vi "data_process.vi"(0 "文件（使用对话框）":path) -> (19 "SENSOR 9":dbl[](array[numeric]), 20 "SENSOR1":dbl[](array[numeric]), 21 "SENSOR 2":dbl[](array[numeric]), 22 "SENSOR 3":dbl[](array[numeric]), 23 "SENSOR 4":dbl[](array[numeric]), 24 "SENSOR 5":dbl[](array[numeric]), 25 "SENSOR 6":dbl[](array[numeric]), 26 "SENSOR 7":dbl[](array[numeric]), 27 "SENSOR 8":dbl[](array[numeric]))   [LabVIEW 2017]
panel:
  out "PWM19":dbl[](array[numeric])
  out "PWM18":dbl[](array[numeric])
  out "PWM17":dbl[](array[numeric])
  out "PWM16":dbl[](array[numeric])
  out "PWM15":dbl[](array[numeric])
  out "PWM14":dbl[](array[numeric])
  out "PWM13":dbl[](array[numeric])
  out "PWM12":dbl[](array[numeric])
  out "PWM11":dbl[](array[numeric])
  out "PWM10":dbl[](array[numeric])
  out "PWM9":dbl[](array[numeric])
  out "PWM8":dbl[](array[numeric])
  out "PWM7":dbl[](array[numeric])
  out "PWM6":dbl[](array[numeric])
  out "PWM5":dbl[](array[numeric])
  out "PWM4":dbl[](array[numeric])
  out "PWM3":dbl[](array[numeric])
  out "匹配偏移量":i32
  out "PWM2":dbl[](array[numeric])
  out "文本":string
  out "PWM1":dbl[](array[numeric])
  # "主要功能：将9行数据分别提取出来作为一个列表"
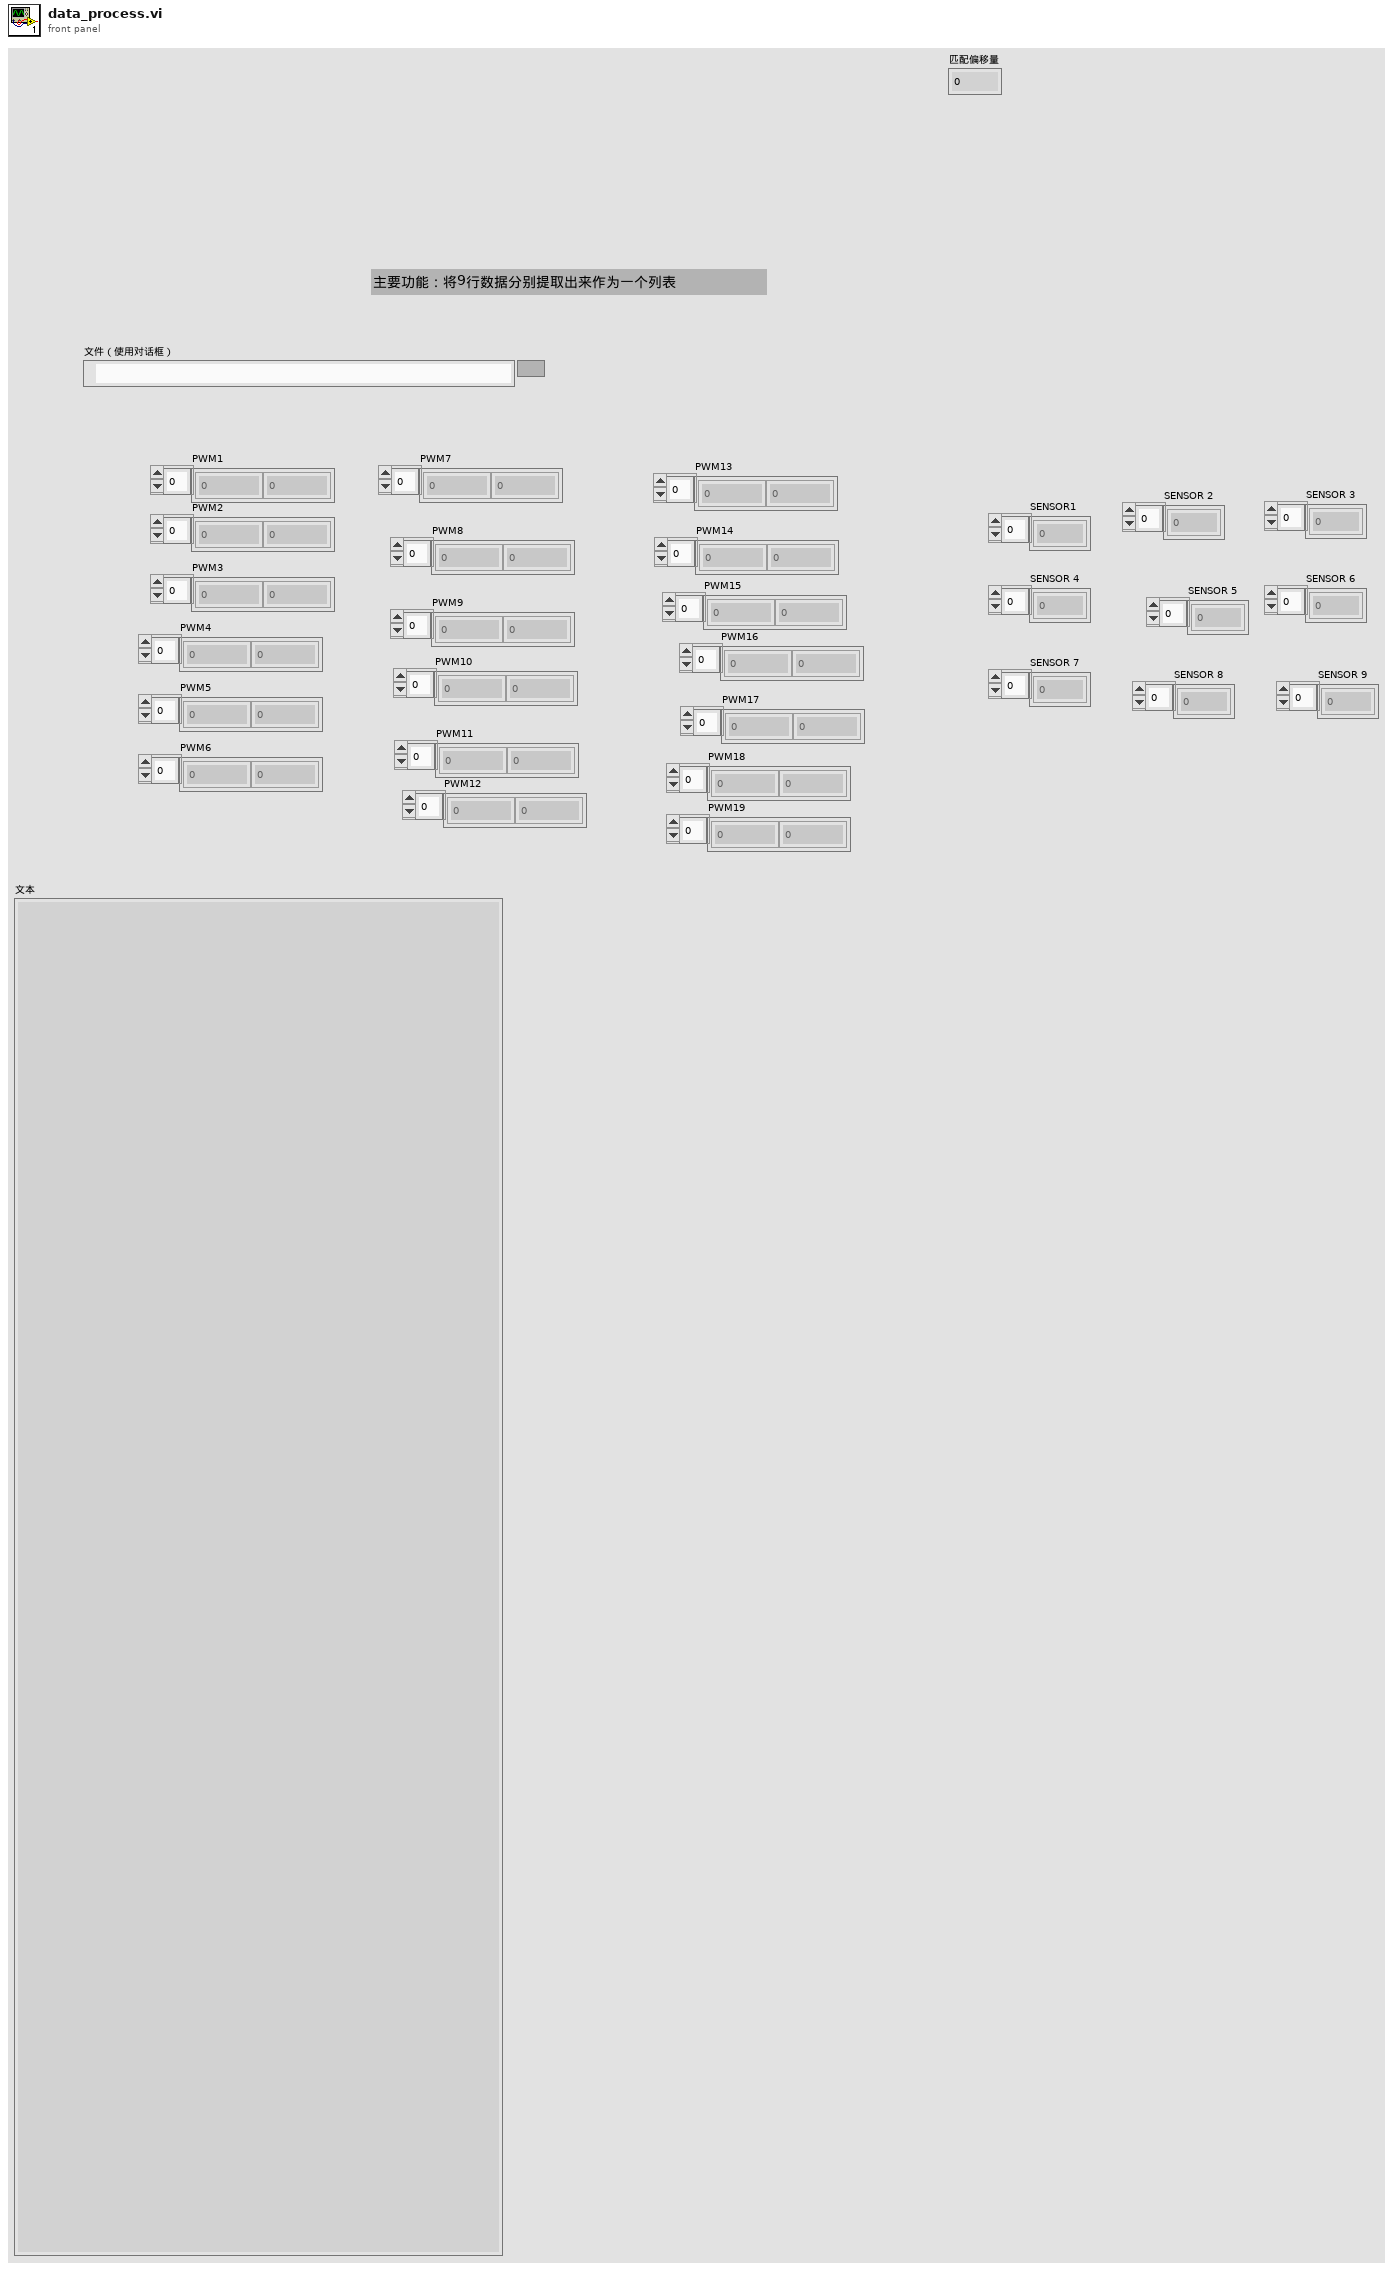
[diagram p1: front panel]
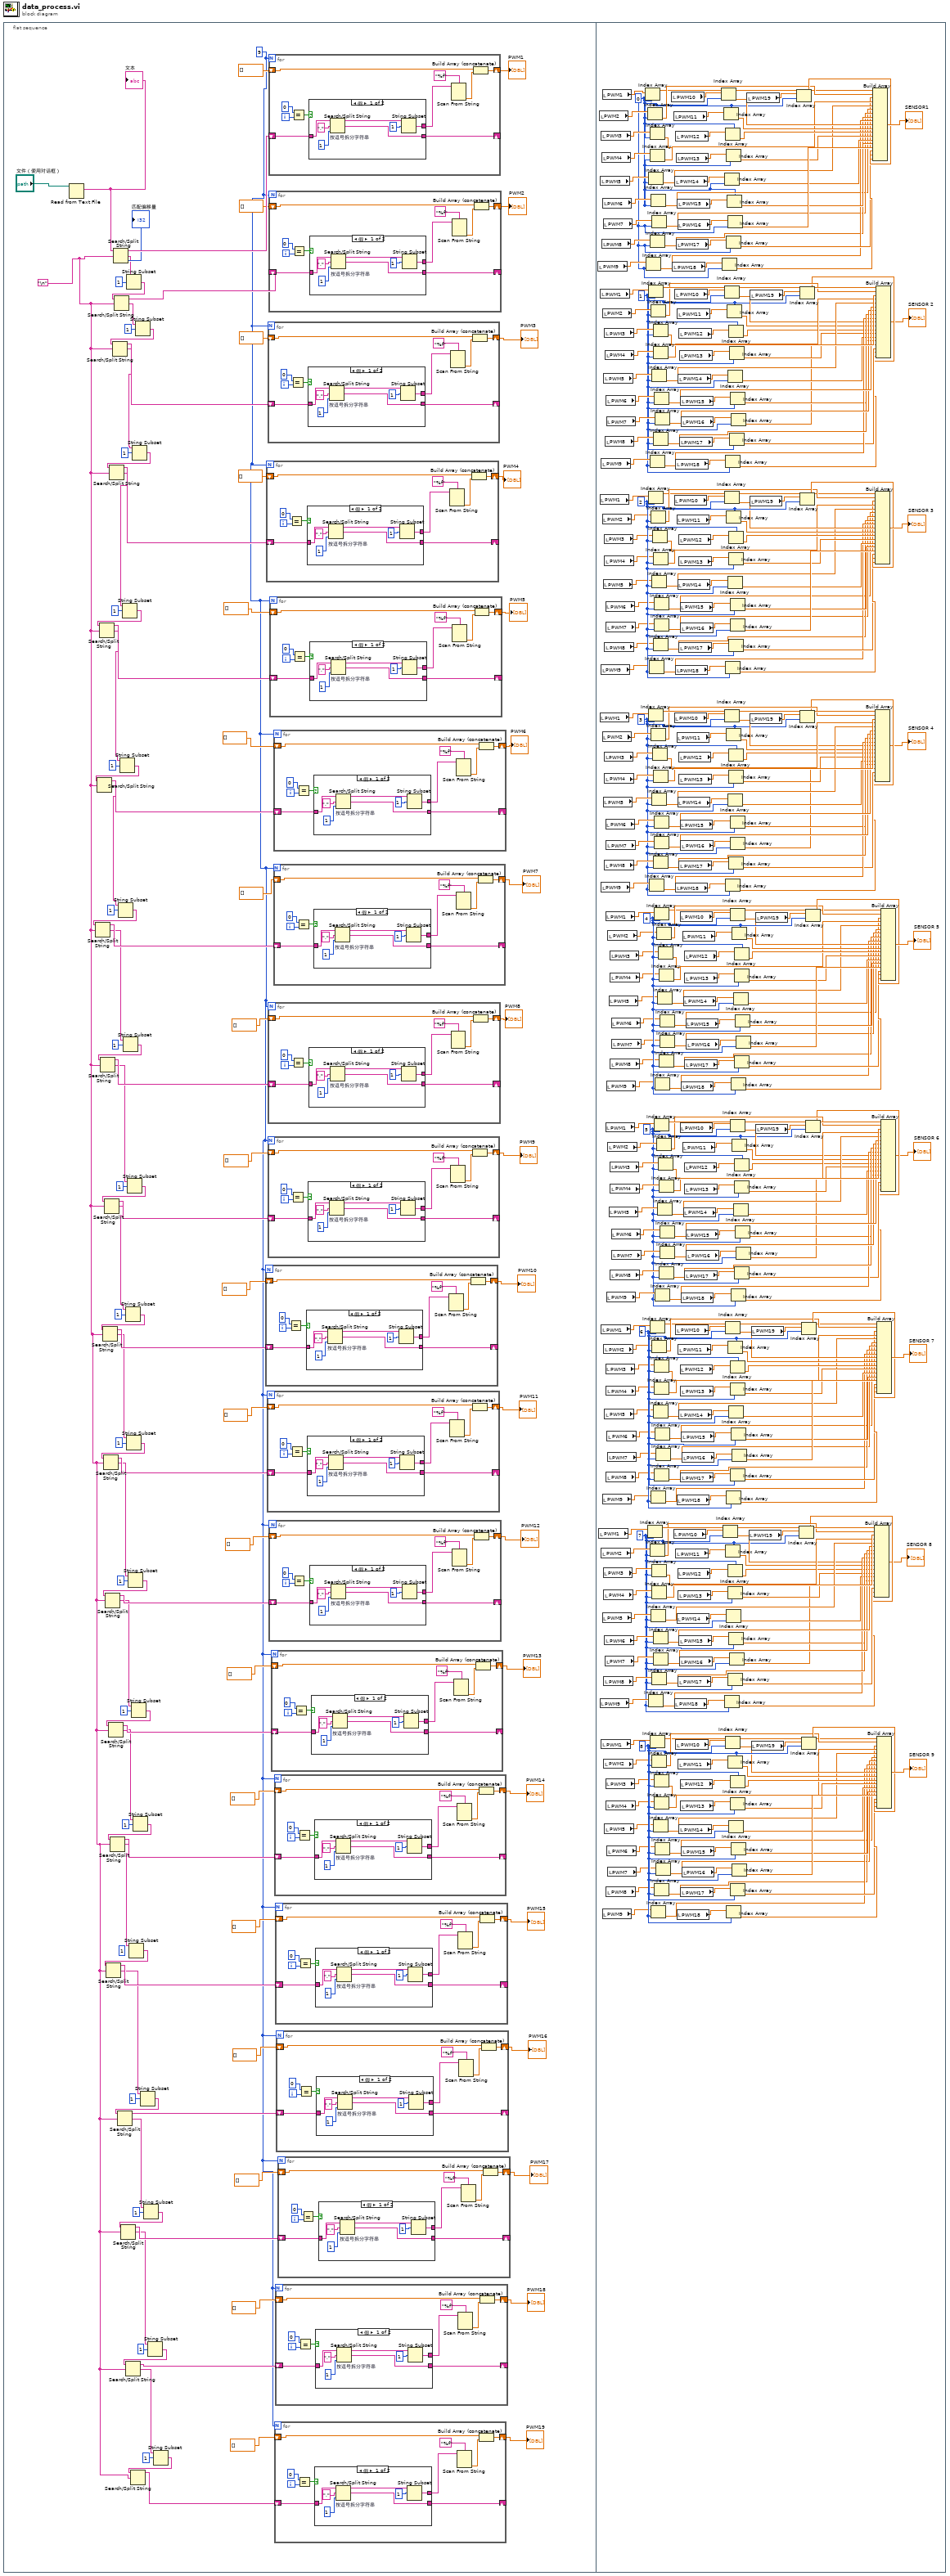
[diagram p0: block diagram]
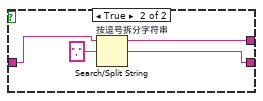
[diagram p2: hidden frame]
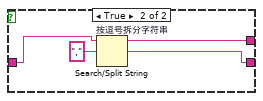
[diagram p3: hidden frame]
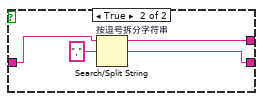
[diagram p4: hidden frame]
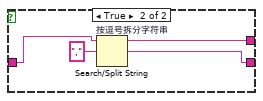
[diagram p5: hidden frame]
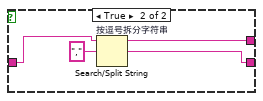
[diagram p6: hidden frame]
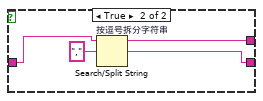
[diagram p7: hidden frame]
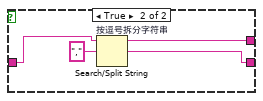
[diagram p8: hidden frame]
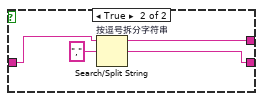
[diagram p9: hidden frame]
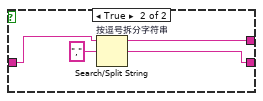
[diagram p10: hidden frame]
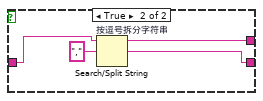
[diagram p11: hidden frame]
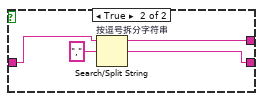
[diagram p12: hidden frame]
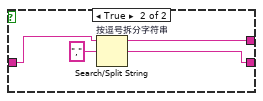
[diagram p13: hidden frame]
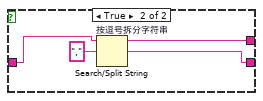
[diagram p14: hidden frame]
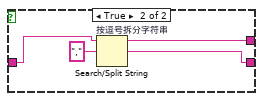
[diagram p15: hidden frame]
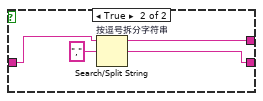
[diagram p16: hidden frame]
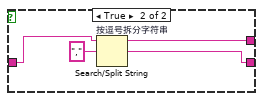
[diagram p17: hidden frame]
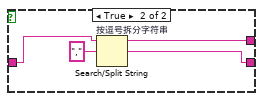
[diagram p18: hidden frame]
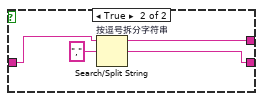
[diagram p19: hidden frame]
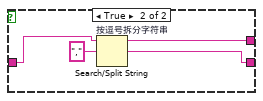
[diagram p20: hidden frame]
diagram:
  n1 = flat-sequence {
    frame #0 {
      (unwired) 1 ("偏移量(0)")
      w4 = "\n"
      w1 = 9
      n2 = Read from Text File(file (use dialog)="文件（使用对话框）") -> (text=w109:string)  [unwired: 3 in, 3 out]
      "文本" <- w109
      n3 = Search/Split String(string=w109, search string/char (-)=w4) -> (substring before match=w112:string, match + rest of string=w106:string, offset of match=→"匹配偏移量":i32)  [unwired: 1 in]
      n4 = String Subset(string=w106, offset (0)=1 ("偏移量(0)")) -> (substring=w105:string)  [unwired: 1 in]
      n5 = Search/Split String(string=w105, search string/char (-)=w4) -> (substring before match=w108:string, match + rest of string=w102:string)  [unwired: 1 in, 1 out]
      n6 = String Subset(string=w102, offset (0)=1 ("偏移量(0)")) -> (substring=w101:string)  [unwired: 1 in]
      n7 = Search/Split String(string=w101, search string/char (-)=w4) -> (substring before match=w100:string, match + rest of string=w80:string)  [unwired: 1 in, 1 out]
      n8 = String Subset(string=w80, offset (0)=1 ("偏移量(0)")) -> (substring=w84:string)  [unwired: 1 in]
      n9 = Search/Split String(string=w84, search string/char (-)=w4) -> (substring before match=w83:string, match + rest of string=w79:string)  [unwired: 1 in, 1 out]
      n10 = String Subset(string=w79, offset (0)=1 ("偏移量(0)")) -> (substring=w81:string)  [unwired: 1 in]
      n11 = Search/Split String(string=w81, search string/char (-)=w4) -> (substring before match=w78:string, match + rest of string=w75:string)  [unwired: 1 in, 1 out]
      n12 = String Subset(string=w75, offset (0)=1 ("偏移量(0)")) -> (substring=w76:string)  [unwired: 1 in]
      n13 = Search/Split String(string=w76, search string/char (-)=w4) -> (substring before match=w74:string, match + rest of string=w71:string)  [unwired: 1 in, 1 out]
      n14 = String Subset(string=w71, offset (0)=1 ("偏移量(0)")) -> (substring=w72:string)  [unwired: 1 in]
      n15 = Search/Split String(string=w72, search string/char (-)=w4) -> (substring before match=w70:string, match + rest of string=w67:string)  [unwired: 1 in, 1 out]
      n16 = String Subset(string=w67, offset (0)=1 ("偏移量(0)")) -> (substring=w68:string)  [unwired: 1 in]
      n17 = Search/Split String(string=w68, search string/char (-)=w4) -> (substring before match=w66:string, match + rest of string=w63:string)  [unwired: 1 in, 1 out]
      n18 = String Subset(string=w63, offset (0)=1 ("偏移量(0)")) -> (substring=w64:string)  [unwired: 1 in]
      n19 = Search/Split String(string=w64, search string/char (-)=w4) -> (substring before match=w62:string, match + rest of string=w40:string)  [unwired: 1 in, 1 out]
      n20 = String Subset(string=w40, offset (0)=1 ("偏移量(0)")) -> (substring=w42:string)  [unwired: 1 in]
      n21 = Search/Split String(string=w42, search string/char (-)=w4) -> (substring before match=w41:string, match + rest of string=w37:string)  [unwired: 1 in, 1 out]
      n22 = String Subset(string=w37, offset (0)=1 ("偏移量(0)")) -> (substring=w38:string)  [unwired: 1 in]
      n23 = Search/Split String(string=w38, search string/char (-)=w4) -> (substring before match=w36:string, match + rest of string=w33:string)  [unwired: 1 in, 1 out]
      n24 = String Subset(string=w33, offset (0)=1 ("偏移量(0)")) -> (substring=w34:string)  [unwired: 1 in]
      n25 = Search/Split String(string=w34, search string/char (-)=w4) -> (substring before match=w32:string, match + rest of string=w30:string)  [unwired: 1 in, 1 out]
      n26 = String Subset(string=w30, offset (0)=1 ("偏移量(0)")) -> (substring=w29:string)  [unwired: 1 in]
      n27 = Search/Split String(string=w29, search string/char (-)=w4) -> (substring before match=w26:string, match + rest of string=w25:string)  [unwired: 1 in, 1 out]
      n28 = String Subset(string=w25, offset (0)=1 ("偏移量(0)")) -> (substring=w27:string)  [unwired: 1 in]
      n29 = Search/Split String(string=w27, search string/char (-)=w4) -> (substring before match=w24:string, match + rest of string=w22:string)  [unwired: 1 in, 1 out]
      n30 = String Subset(string=w22) -> (substring=w23:string)  [unwired: 2 in]
      n31 = Search/Split String(string=w23, search string/char (-)=w4) -> (substring before match=w21:string, match + rest of string=w18:string)  [unwired: 1 in, 1 out]
      n32 = String Subset(string=w18, offset (0)=1 ("偏移量(0)")) -> (substring=w19:string)  [unwired: 1 in]
      n33 = Search/Split String(string=w19, search string/char (-)=w4) -> (substring before match=w17:string, match + rest of string=w14:string)  [unwired: 1 in, 1 out]
      n34 = String Subset(string=w14, offset (0)=1 ("偏移量(0)")) -> (substring=w15:string)  [unwired: 1 in]
      n35 = Search/Split String(string=w15, search string/char (-)=w4) -> (substring before match=w13:string, match + rest of string=w10:string)  [unwired: 1 in, 1 out]
      n36 = String Subset(string=w10, offset (0)=1 ("偏移量(0)")) -> (substring=w11:string)  [unwired: 1 in]
      n37 = Search/Split String(string=w11, search string/char (-)=w4) -> (substring before match=w9:string, match + rest of string=w3:string)  [unwired: 1 in, 1 out]
      n38 = String Subset(string=w3, offset (0)=1 ("偏移量(0)")) -> (substring=w5:string)  [unwired: 1 in]
      n39 = Search/Split String(string=w5, search string/char (-)=w4) -> (substring before match=w2:string)  [unwired: 1 in, 2 out]
      n40 = for {
        N: w1 -> [_]
        shift-right: [w310] -> _
        shift-left: w41 -> [w311]
        shift-right: [w307] -> w61
        shift-left: dbl[] [] -> [w305]
        i -> [w314]
        n41 = Equal?(x=0, y=w314) -> (x = y?=w312:bool)
        n42 = case shown="假" w312 {
          tunnel: [w320 w324] -> w310
          tunnel: w311 -> [w321 w323]
          tunnel: [w315 w322] -> w308
          frame False {
            n43 = Search/Split String "按逗号拆分字符串"(string=w321, search string/char (-)="," ("搜索字符串/字符(-)"), offset (0)=1 ("偏移量(0)")) -> (substring before match=w317:string, match + rest of string=w320:string)  [unwired: 1 out]
            n44 = String Subset(string=w317, offset (0)=1 ("偏移量(0)")) -> (substring=w315:string)  [unwired: 1 in]
          }
          frame True {
            n45 = Search/Split String "按逗号拆分字符串"(string=w323, search string/char (-)="," ("搜索字符串/字符(-)")) -> (substring before match=w322:string, match + rest of string=w324:string)  [unwired: 1 in, 1 out]
          }
        }
        n46 = Scan From String(format string="%f" ("格式字符串"), input string=w308) -> (output 1=w306:dbl)  [unwired: 3 in, 3 out]
        n47 = Build Array (concatenate)(w305, w306) -> (w307:dbl[])
      }
      "PWM10" <- w61
      n48 = for {
        N: w1 -> [_]
        shift-right: [w436] -> _
        shift-left: w83 -> [w437]
        shift-right: [w433] -> w97
        shift-left: dbl[] [] -> [w431]
        i -> [w440]
        n49 = Equal?(x=0, y=w440) -> (x = y?=w438:bool)
        n50 = case shown="假" w438 {
          tunnel: [w446 w450] -> w436
          tunnel: w437 -> [w447 w449]
          tunnel: [w441 w448] -> w434
          frame False {
            n51 = Search/Split String "按逗号拆分字符串"(string=w447, search string/char (-)="," ("搜索字符串/字符(-)"), offset (0)=1 ("偏移量(0)")) -> (substring before match=w443:string, match + rest of string=w446:string)  [unwired: 1 out]
            n52 = String Subset(string=w443, offset (0)=1 ("偏移量(0)")) -> (substring=w441:string)  [unwired: 1 in]
          }
          frame True {
            n53 = Search/Split String "按逗号拆分字符串"(string=w449, search string/char (-)="," ("搜索字符串/字符(-)")) -> (substring before match=w448:string, match + rest of string=w450:string)  [unwired: 1 in, 1 out]
          }
        }
        n54 = Scan From String(format string="%f" ("格式字符串"), input string=w434) -> (output 1=w432:dbl)  [unwired: 3 in, 3 out]
        n55 = Build Array (concatenate)(w431, w432) -> (w433:dbl[])
      }
      "PWM4" <- w97
      n56 = for {
        N: w1 -> [_]
        shift-right: [w289] -> _
        shift-left: w36 -> [w290]
        shift-right: [w286] -> w59
        shift-left: dbl[] [] -> [w284]
        i -> [w293]
        n57 = Equal?(x=0, y=w293) -> (x = y?=w291:bool)
        n58 = case shown="假" w291 {
          tunnel: [w299 w303] -> w289
          tunnel: w290 -> [w300 w302]
          tunnel: [w294 w301] -> w287
          frame False {
            n59 = Search/Split String "按逗号拆分字符串"(string=w300, search string/char (-)="," ("搜索字符串/字符(-)"), offset (0)=1 ("偏移量(0)")) -> (substring before match=w296:string, match + rest of string=w299:string)  [unwired: 1 out]
            n60 = String Subset(string=w296, offset (0)=1 ("偏移量(0)")) -> (substring=w294:string)  [unwired: 1 in]
          }
          frame True {
            n61 = Search/Split String "按逗号拆分字符串"(string=w302, search string/char (-)="," ("搜索字符串/字符(-)")) -> (substring before match=w301:string, match + rest of string=w303:string)  [unwired: 1 in, 1 out]
          }
        }
        n62 = Scan From String(format string="%f" ("格式字符串"), input string=w287) -> (output 1=w285:dbl)  [unwired: 3 in, 3 out]
        n63 = Build Array (concatenate)(w284, w285) -> (w286:dbl[])
      }
      "PWM11" <- w59
      n64 = for {
        N: w1 -> [_]
        shift-right: [w457] -> _
        shift-left: w100 -> [w458]
        shift-right: [w454] -> w98
        shift-left: dbl[] [] -> [w452]
        i -> [w461]
        n65 = Equal?(x=0, y=w461) -> (x = y?=w459:bool)
        n66 = case shown="假" w459 {
          tunnel: [w467 w471] -> w457
          tunnel: w458 -> [w468 w470]
          tunnel: [w462 w469] -> w455
          frame False {
            n67 = Search/Split String "按逗号拆分字符串"(string=w468, search string/char (-)="," ("搜索字符串/字符(-)"), offset (0)=1 ("偏移量(0)")) -> (substring before match=w464:string, match + rest of string=w467:string)  [unwired: 1 out]
            n68 = String Subset(string=w464, offset (0)=1 ("偏移量(0)")) -> (substring=w462:string)  [unwired: 1 in]
          }
          frame True {
            n69 = Search/Split String "按逗号拆分字符串"(string=w470, search string/char (-)="," ("搜索字符串/字符(-)")) -> (substring before match=w469:string, match + rest of string=w471:string)  [unwired: 1 in, 1 out]
          }
        }
        n70 = Scan From String(format string="%f" ("格式字符串"), input string=w455) -> (output 1=w453:dbl)  [unwired: 3 in, 3 out]
        n71 = Build Array (concatenate)(w452, w453) -> (w454:dbl[])
      }
      "PWM3" <- w98
      n72 = for {
        N: w1 -> [_]
        shift-right: [w331] -> _
        shift-left: w62 -> [w332]
        shift-right: [w328] -> w92
        shift-left: dbl[] [] -> [w326]
        i -> [w335]
        n73 = Equal?(x=0, y=w335) -> (x = y?=w333:bool)
        n74 = case shown="假" w333 {
          tunnel: [w341 w345] -> w331
          tunnel: w332 -> [w342 w344]
          tunnel: [w336 w343] -> w329
          frame False {
            n75 = Search/Split String "按逗号拆分字符串"(string=w342, search string/char (-)="," ("搜索字符串/字符(-)"), offset (0)=1 ("偏移量(0)")) -> (substring before match=w338:string, match + rest of string=w341:string)  [unwired: 1 out]
            n76 = String Subset(string=w338, offset (0)=1 ("偏移量(0)")) -> (substring=w336:string)  [unwired: 1 in]
          }
          frame True {
            n77 = Search/Split String "按逗号拆分字符串"(string=w344, search string/char (-)="," ("搜索字符串/字符(-)")) -> (substring before match=w343:string, match + rest of string=w345:string)  [unwired: 1 in, 1 out]
          }
        }
        n78 = Scan From String(format string="%f" ("格式字符串"), input string=w329) -> (output 1=w327:dbl)  [unwired: 3 in, 3 out]
        n79 = Build Array (concatenate)(w326, w327) -> (w328:dbl[])
      }
      "PWM9" <- w92
      n80 = for {
        N: w1 -> [_]
        shift-right: [w352] -> _
        shift-left: w66 -> [w353]
        shift-right: [w349] -> w93
        shift-left: dbl[] [] -> [w347]
        i -> [w356]
        n81 = Equal?(x=0, y=w356) -> (x = y?=w354:bool)
        n82 = case shown="假" w354 {
          tunnel: [w362 w366] -> w352
          tunnel: w353 -> [w363 w365]
          tunnel: [w357 w364] -> w350
          frame False {
            n83 = Search/Split String "按逗号拆分字符串"(string=w363, search string/char (-)="," ("搜索字符串/字符(-)"), offset (0)=1 ("偏移量(0)")) -> (substring before match=w359:string, match + rest of string=w362:string)  [unwired: 1 out]
            n84 = String Subset(string=w359, offset (0)=1 ("偏移量(0)")) -> (substring=w357:string)  [unwired: 1 in]
          }
          frame True {
            n85 = Search/Split String "按逗号拆分字符串"(string=w365, search string/char (-)="," ("搜索字符串/字符(-)")) -> (substring before match=w364:string, match + rest of string=w366:string)  [unwired: 1 in, 1 out]
          }
        }
        n86 = Scan From String(format string="%f" ("格式字符串"), input string=w350) -> (output 1=w348:dbl)  [unwired: 3 in, 3 out]
        n87 = Build Array (concatenate)(w347, w348) -> (w349:dbl[])
      }
      "PWM8" <- w93
      n88 = for {
        N: w1 -> [_]
        shift-right: [w499] -> _
        shift-left: w112 -> [w500]
        shift-right: [w496] -> w113
        shift-left: dbl[] [] -> [w494]
        i -> [w503]
        n89 = Equal?(x=0, y=w503) -> (x = y?=w501:bool)
        n90 = case shown="假" w501 {
          tunnel: [w509 w513] -> w499
          tunnel: w500 -> [w510 w512]
          tunnel: [w504 w511] -> w497
          frame False {
            n91 = Search/Split String "按逗号拆分字符串"(string=w510, search string/char (-)="," ("搜索字符串/字符(-)"), offset (0)=1 ("偏移量(0)")) -> (substring before match=w506:string, match + rest of string=w509:string)  [unwired: 1 out]
            n92 = String Subset(string=w506, offset (0)=1 ("偏移量(0)")) -> (substring=w504:string)  [unwired: 1 in]
          }
          frame True {
            n93 = Search/Split String "按逗号拆分字符串"(string=w512, search string/char (-)="," ("搜索字符串/字符(-)")) -> (substring before match=w511:string, match + rest of string=w513:string)  [unwired: 1 in, 1 out]
          }
        }
        n94 = Scan From String(format string="%f" ("格式字符串"), input string=w497) -> (output 1=w495:dbl)  [unwired: 3 in, 3 out]
        n95 = Build Array (concatenate)(w494, w495) -> (w496:dbl[])
      }
      "PWM1" <- w113
      n96 = for {
        N: w1 -> [_]
        shift-right: [w478] -> _
        shift-left: w108 -> [w479]
        shift-right: [w475] -> w110
        shift-left: dbl[] [] -> [w473]
        i -> [w482]
        n97 = Equal?(x=0, y=w482) -> (x = y?=w480:bool)
        n98 = case shown="假" w480 {
          tunnel: [w488 w492] -> w478
          tunnel: w479 -> [w489 w491]
          tunnel: [w483 w490] -> w476
          frame False {
            n99 = Search/Split String "按逗号拆分字符串"(string=w489, search string/char (-)="," ("搜索字符串/字符(-)"), offset (0)=1 ("偏移量(0)")) -> (substring before match=w485:string, match + rest of string=w488:string)  [unwired: 1 out]
            n100 = String Subset(string=w485, offset (0)=1 ("偏移量(0)")) -> (substring=w483:string)  [unwired: 1 in]
          }
          frame True {
            n101 = Search/Split String "按逗号拆分字符串"(string=w491, search string/char (-)="," ("搜索字符串/字符(-)")) -> (substring before match=w490:string, match + rest of string=w492:string)  [unwired: 1 in, 1 out]
          }
        }
        n102 = Scan From String(format string="%f" ("格式字符串"), input string=w476) -> (output 1=w474:dbl)  [unwired: 3 in, 3 out]
        n103 = Build Array (concatenate)(w473, w474) -> (w475:dbl[])
      }
      "PWM2" <- w110
      n104 = for {
        N: w1 -> [_]
        shift-right: [w268] -> _
        shift-left: w32 -> [w269]
        shift-right: [w265] -> w57
        shift-left: dbl[] [] -> [w263]
        i -> [w272]
        n105 = Equal?(x=0, y=w272) -> (x = y?=w270:bool)
        n106 = case shown="假" w270 {
          tunnel: [w278 w282] -> w268
          tunnel: w269 -> [w279 w281]
          tunnel: [w273 w280] -> w266
          frame False {
            n107 = Search/Split String "按逗号拆分字符串"(string=w279, search string/char (-)="," ("搜索字符串/字符(-)"), offset (0)=1 ("偏移量(0)")) -> (substring before match=w275:string, match + rest of string=w278:string)  [unwired: 1 out]
            n108 = String Subset(string=w275, offset (0)=1 ("偏移量(0)")) -> (substring=w273:string)  [unwired: 1 in]
          }
          frame True {
            n109 = Search/Split String "按逗号拆分字符串"(string=w281, search string/char (-)="," ("搜索字符串/字符(-)")) -> (substring before match=w280:string, match + rest of string=w282:string)  [unwired: 1 in, 1 out]
          }
        }
        n110 = Scan From String(format string="%f" ("格式字符串"), input string=w266) -> (output 1=w264:dbl)  [unwired: 3 in, 3 out]
        n111 = Build Array (concatenate)(w263, w264) -> (w265:dbl[])
      }
      "PWM12" <- w57
      n112 = for {
        N: w1 -> [_]
        shift-right: [w415] -> _
        shift-left: w78 -> [w416]
        shift-right: [w412] -> w96
        shift-left: dbl[] [] -> [w410]
        i -> [w419]
        n113 = Equal?(x=0, y=w419) -> (x = y?=w417:bool)
        n114 = case shown="假" w417 {
          tunnel: [w425 w429] -> w415
          tunnel: w416 -> [w426 w428]
          tunnel: [w420 w427] -> w413
          frame False {
            n115 = Search/Split String "按逗号拆分字符串"(string=w426, search string/char (-)="," ("搜索字符串/字符(-)"), offset (0)=1 ("偏移量(0)")) -> (substring before match=w422:string, match + rest of string=w425:string)  [unwired: 1 out]
            n116 = String Subset(string=w422, offset (0)=1 ("偏移量(0)")) -> (substring=w420:string)  [unwired: 1 in]
          }
          frame True {
            n117 = Search/Split String "按逗号拆分字符串"(string=w428, search string/char (-)="," ("搜索字符串/字符(-)")) -> (substring before match=w427:string, match + rest of string=w429:string)  [unwired: 1 in, 1 out]
          }
        }
        n118 = Scan From String(format string="%f" ("格式字符串"), input string=w413) -> (output 1=w411:dbl)  [unwired: 3 in, 3 out]
        n119 = Build Array (concatenate)(w410, w411) -> (w412:dbl[])
      }
      "PWM5" <- w96
      n120 = for {
        N: w1 -> [_]
        shift-right: [w247] -> _
        shift-left: w26 -> [w248]
        shift-right: [w244] -> w55
        shift-left: dbl[] [] -> [w242]
        i -> [w251]
        n121 = Equal?(x=0, y=w251) -> (x = y?=w249:bool)
        n122 = case shown="假" w249 {
          tunnel: [w257 w261] -> w247
          tunnel: w248 -> [w258 w260]
          tunnel: [w252 w259] -> w245
          frame False {
            n123 = Search/Split String "按逗号拆分字符串"(string=w258, search string/char (-)="," ("搜索字符串/字符(-)"), offset (0)=1 ("偏移量(0)")) -> (substring before match=w254:string, match + rest of string=w257:string)  [unwired: 1 out]
            n124 = String Subset(string=w254, offset (0)=1 ("偏移量(0)")) -> (substring=w252:string)  [unwired: 1 in]
          }
          frame True {
            n125 = Search/Split String "按逗号拆分字符串"(string=w260, search string/char (-)="," ("搜索字符串/字符(-)")) -> (substring before match=w259:string, match + rest of string=w261:string)  [unwired: 1 in, 1 out]
          }
        }
        n126 = Scan From String(format string="%f" ("格式字符串"), input string=w245) -> (output 1=w243:dbl)  [unwired: 3 in, 3 out]
        n127 = Build Array (concatenate)(w242, w243) -> (w244:dbl[])
      }
      "PWM13" <- w55
      n128 = for {
        N: w1 -> [_]
        shift-right: [w373] -> _
        shift-left: w70 -> [w374]
        shift-right: [w370] -> w94
        shift-left: dbl[] [] -> [w368]
        i -> [w377]
        n129 = Equal?(x=0, y=w377) -> (x = y?=w375:bool)
        n130 = case shown="假" w375 {
          tunnel: [w383 w387] -> w373
          tunnel: w374 -> [w384 w386]
          tunnel: [w378 w385] -> w371
          frame False {
            n131 = Search/Split String "按逗号拆分字符串"(string=w384, search string/char (-)="," ("搜索字符串/字符(-)"), offset (0)=1 ("偏移量(0)")) -> (substring before match=w380:string, match + rest of string=w383:string)  [unwired: 1 out]
            n132 = String Subset(string=w380, offset (0)=1 ("偏移量(0)")) -> (substring=w378:string)  [unwired: 1 in]
          }
          frame True {
            n133 = Search/Split String "按逗号拆分字符串"(string=w386, search string/char (-)="," ("搜索字符串/字符(-)")) -> (substring before match=w385:string, match + rest of string=w387:string)  [unwired: 1 in, 1 out]
          }
        }
        n134 = Scan From String(format string="%f" ("格式字符串"), input string=w371) -> (output 1=w369:dbl)  [unwired: 3 in, 3 out]
        n135 = Build Array (concatenate)(w368, w369) -> (w370:dbl[])
      }
      "PWM7" <- w94
      n136 = for {
        N: w1 -> [_]
        shift-right: [w394] -> _
        shift-left: w74 -> [w395]
        shift-right: [w391] -> w95
        shift-left: dbl[] [] -> [w389]
        i -> [w398]
        n137 = Equal?(x=0, y=w398) -> (x = y?=w396:bool)
        n138 = case shown="假" w396 {
          tunnel: [w404 w408] -> w394
          tunnel: w395 -> [w405 w407]
          tunnel: [w399 w406] -> w392
          frame False {
            n139 = Search/Split String "按逗号拆分字符串"(string=w405, search string/char (-)="," ("搜索字符串/字符(-)"), offset (0)=1 ("偏移量(0)")) -> (substring before match=w401:string, match + rest of string=w404:string)  [unwired: 1 out]
            n140 = String Subset(string=w401, offset (0)=1 ("偏移量(0)")) -> (substring=w399:string)  [unwired: 1 in]
          }
          frame True {
            n141 = Search/Split String "按逗号拆分字符串"(string=w407, search string/char (-)="," ("搜索字符串/字符(-)")) -> (substring before match=w406:string, match + rest of string=w408:string)  [unwired: 1 in, 1 out]
          }
        }
        n142 = Scan From String(format string="%f" ("格式字符串"), input string=w392) -> (output 1=w390:dbl)  [unwired: 3 in, 3 out]
        n143 = Build Array (concatenate)(w389, w390) -> (w391:dbl[])
      }
      "PWM6" <- w95
      n144 = for {
        N: w1 -> [_]
        shift-right: [w226] -> _
        shift-left: w24 -> [w227]
        shift-right: [w223] -> w53
        shift-left: dbl[] [] -> [w221]
        i -> [w230]
        n145 = Equal?(x=0, y=w230) -> (x = y?=w228:bool)
        n146 = case shown="假" w228 {
          tunnel: [w236 w240] -> w226
          tunnel: w227 -> [w237 w239]
          tunnel: [w231 w238] -> w224
          frame False {
            n147 = Search/Split String "按逗号拆分字符串"(string=w237, search string/char (-)="," ("搜索字符串/字符(-)"), offset (0)=1 ("偏移量(0)")) -> (substring before match=w233:string, match + rest of string=w236:string)  [unwired: 1 out]
            n148 = String Subset(string=w233, offset (0)=1 ("偏移量(0)")) -> (substring=w231:string)  [unwired: 1 in]
          }
          frame True {
            n149 = Search/Split String "按逗号拆分字符串"(string=w239, search string/char (-)="," ("搜索字符串/字符(-)")) -> (substring before match=w238:string, match + rest of string=w240:string)  [unwired: 1 in, 1 out]
          }
        }
        n150 = Scan From String(format string="%f" ("格式字符串"), input string=w224) -> (output 1=w222:dbl)  [unwired: 3 in, 3 out]
        n151 = Build Array (concatenate)(w221, w222) -> (w223:dbl[])
      }
      "PWM14" <- w53
      n152 = for {
        N: w1 -> [_]
        shift-right: [w121] -> _
        shift-left: w2 -> [w122]
        shift-right: [w118] -> w8
        shift-left: dbl[] [] -> [w116]
        i -> [w125]
        n153 = Equal?(x=0, y=w125) -> (x = y?=w123:bool)
        n154 = case shown="假" w123 {
          tunnel: [w131 w135] -> w121
          tunnel: w122 -> [w132 w134]
          tunnel: [w126 w133] -> w119
          frame False {
            n155 = Search/Split String "按逗号拆分字符串"(string=w132, search string/char (-)="," ("搜索字符串/字符(-)"), offset (0)=1 ("偏移量(0)")) -> (substring before match=w128:string, match + rest of string=w131:string)  [unwired: 1 out]
            n156 = String Subset(string=w128, offset (0)=1 ("偏移量(0)")) -> (substring=w126:string)  [unwired: 1 in]
          }
          frame True {
            n157 = Search/Split String "按逗号拆分字符串"(string=w134, search string/char (-)="," ("搜索字符串/字符(-)")) -> (substring before match=w133:string, match + rest of string=w135:string)  [unwired: 1 in, 1 out]
          }
        }
        n158 = Scan From String(format string="%f" ("格式字符串"), input string=w119) -> (output 1=w117:dbl)  [unwired: 3 in, 3 out]
        n159 = Build Array (concatenate)(w116, w117) -> (w118:dbl[])
      }
      "PWM19" <- w8
      n160 = for {
        N: w1 -> [_]
        shift-right: [w205] -> _
        shift-left: w21 -> [w206]
        shift-right: [w202] -> w51
        shift-left: dbl[] [] -> [w200]
        i -> [w209]
        n161 = Equal?(x=0, y=w209) -> (x = y?=w207:bool)
        n162 = case shown="假" w207 {
          tunnel: [w215 w219] -> w205
          tunnel: w206 -> [w216 w218]
          tunnel: [w210 w217] -> w203
          frame False {
            n163 = Search/Split String "按逗号拆分字符串"(string=w216, search string/char (-)="," ("搜索字符串/字符(-)"), offset (0)=1 ("偏移量(0)")) -> (substring before match=w212:string, match + rest of string=w215:string)  [unwired: 1 out]
            n164 = String Subset(string=w212, offset (0)=1 ("偏移量(0)")) -> (substring=w210:string)  [unwired: 1 in]
          }
          frame True {
            n165 = Search/Split String "按逗号拆分字符串"(string=w218, search string/char (-)="," ("搜索字符串/字符(-)")) -> (substring before match=w217:string, match + rest of string=w219:string)  [unwired: 1 in, 1 out]
          }
        }
        n166 = Scan From String(format string="%f" ("格式字符串"), input string=w203) -> (output 1=w201:dbl)  [unwired: 3 in, 3 out]
        n167 = Build Array (concatenate)(w200, w201) -> (w202:dbl[])
      }
      "PWM15" <- w51
      n168 = for {
        N: w1 -> [_]
        shift-right: [w142] -> _
        shift-left: w9 -> [w143]
        shift-right: [w139] -> w45
        shift-left: dbl[] [] -> [w137]
        i -> [w146]
        n169 = Equal?(x=0, y=w146) -> (x = y?=w144:bool)
        n170 = case shown="假" w144 {
          tunnel: [w152 w156] -> w142
          tunnel: w143 -> [w153 w155]
          tunnel: [w147 w154] -> w140
          frame False {
            n171 = Search/Split String "按逗号拆分字符串"(string=w153, search string/char (-)="," ("搜索字符串/字符(-)"), offset (0)=1 ("偏移量(0)")) -> (substring before match=w149:string, match + rest of string=w152:string)  [unwired: 1 out]
            n172 = String Subset(string=w149, offset (0)=1 ("偏移量(0)")) -> (substring=w147:string)  [unwired: 1 in]
          }
          frame True {
            n173 = Search/Split String "按逗号拆分字符串"(string=w155, search string/char (-)="," ("搜索字符串/字符(-)")) -> (substring before match=w154:string, match + rest of string=w156:string)  [unwired: 1 in, 1 out]
          }
        }
        n174 = Scan From String(format string="%f" ("格式字符串"), input string=w140) -> (output 1=w138:dbl)  [unwired: 3 in, 3 out]
        n175 = Build Array (concatenate)(w137, w138) -> (w139:dbl[])
      }
      "PWM18" <- w45
      n176 = for {
        N: w1 -> [_]
        shift-right: [w184] -> _
        shift-left: w17 -> [w185]
        shift-right: [w181] -> w49
        shift-left: dbl[] [] -> [w179]
        i -> [w188]
        n177 = Equal?(x=0, y=w188) -> (x = y?=w186:bool)
        n178 = case shown="假" w186 {
          tunnel: [w194 w198] -> w184
          tunnel: w185 -> [w195 w197]
          tunnel: [w189 w196] -> w182
          frame False {
            n179 = Search/Split String "按逗号拆分字符串"(string=w195, search string/char (-)="," ("搜索字符串/字符(-)"), offset (0)=1 ("偏移量(0)")) -> (substring before match=w191:string, match + rest of string=w194:string)  [unwired: 1 out]
            n180 = String Subset(string=w191, offset (0)=1 ("偏移量(0)")) -> (substring=w189:string)  [unwired: 1 in]
          }
          frame True {
            n181 = Search/Split String "按逗号拆分字符串"(string=w197, search string/char (-)="," ("搜索字符串/字符(-)")) -> (substring before match=w196:string, match + rest of string=w198:string)  [unwired: 1 in, 1 out]
          }
        }
        n182 = Scan From String(format string="%f" ("格式字符串"), input string=w182) -> (output 1=w180:dbl)  [unwired: 3 in, 3 out]
        n183 = Build Array (concatenate)(w179, w180) -> (w181:dbl[])
      }
      "PWM16" <- w49
      n184 = for {
        N: w1 -> [_]
        shift-right: [w163] -> _
        shift-left: w13 -> [w164]
        shift-right: [w160] -> w47
        shift-left: dbl[] [] -> [w158]
        i -> [w167]
        n185 = Equal?(x=0, y=w167) -> (x = y?=w165:bool)
        n186 = case shown="假" w165 {
          tunnel: [w173 w177] -> w163
          tunnel: w164 -> [w174 w176]
          tunnel: [w168 w175] -> w161
          frame False {
            n187 = Search/Split String "按逗号拆分字符串"(string=w174, search string/char (-)="," ("搜索字符串/字符(-)"), offset (0)=1 ("偏移量(0)")) -> (substring before match=w170:string, match + rest of string=w173:string)  [unwired: 1 out]
            n188 = String Subset(string=w170, offset (0)=1 ("偏移量(0)")) -> (substring=w168:string)  [unwired: 1 in]
          }
          frame True {
            n189 = Search/Split String "按逗号拆分字符串"(string=w176, search string/char (-)="," ("搜索字符串/字符(-)")) -> (substring before match=w175:string, match + rest of string=w177:string)  [unwired: 1 in, 1 out]
          }
        }
        n190 = Scan From String(format string="%f" ("格式字符串"), input string=w161) -> (output 1=w159:dbl)  [unwired: 3 in, 3 out]
        n191 = Build Array (concatenate)(w158, w159) -> (w160:dbl[])
      }
      "PWM17" <- w47
    }
    frame #1 {
      w554 = 8 ("索引")
      w555 = 7 ("索引")
      w634 = 6 ("索引")
      w635 = 5 ("索引")
      w714 = 4 ("索引")
      w715 = 3 ("索引")
      w794 = 2 ("索引")
      w796 = 1 ("索引")
      w795 = 0 ("索引")
      n192 = local read "PWM9"() -> (w805:dbl[])
      n193 = local read "PWM1"() -> (w594:dbl[])
      n194 = local read "PWM2"() -> (w798:dbl[])
      n195 = local read "PWM1"() -> (w755:dbl[])
      n196 = local read "PWM1"() -> (w754:dbl[])
      n197 = local read "PWM9"() -> (w585:dbl[])
      n198 = local read "PWM5"() -> (w801:dbl[])
      n199 = local read "PWM1"() -> (w873:dbl[])
      n200 = local read "PWM9"() -> (w764:dbl[])
      n201 = local read "PWM9"() -> (w745:dbl[])
      n202 = local read "PWM3"() -> (w799:dbl[])
      n203 = local read "PWM9"() -> (w864:dbl[])
      n204 = local read "PWM1"() -> (w595:dbl[])
      n205 = local read "PWM2"() -> (w592:dbl[])
      n206 = local read "PWM1"() -> (w515:dbl[])
      n207 = local read "PWM4"() -> (w800:dbl[])
      n208 = local read "PWM8"() -> (w804:dbl[])
      n209 = local read "PWM1"() -> (w874:dbl[])
      n210 = local read "PWM2"() -> (w757:dbl[])
      n211 = local read "PWM2"() -> (w752:dbl[])
      n212 = local read "PWM9"() -> (w604:dbl[])
      n213 = local read "PWM5"() -> (w589:dbl[])
      n214 = local read "PWM9"() -> (w524:dbl[])
      n215 = local read "PWM6"() -> (w802:dbl[])
      n216 = local read "PWM2"() -> (w871:dbl[])
      n217 = local read "PWM7"() -> (w803:dbl[])
      n218 = local read "PWM5"() -> (w760:dbl[])
      n219 = local read "PWM5"() -> (w749:dbl[])
      n220 = local read "PWM3"() -> (w591:dbl[])
      n221 = local read "PWM5"() -> (w868:dbl[])
      n222 = local read "PWM2"() -> (w597:dbl[])
      n223 = local read "PWM4"() -> (w590:dbl[])
      n224 = local read "PWM8"() -> (w586:dbl[])
      n225 = local read "PWM2"() -> (w517:dbl[])
      n226 = local read "PWM3"() -> (w758:dbl[])
      n227 = local read "PWM3"() -> (w751:dbl[])
      n228 = local read "PWM3"() -> (w870:dbl[])
      n229 = local read "PWM4"() -> (w759:dbl[])
      n230 = local read "PWM8"() -> (w763:dbl[])
      n231 = local read "PWM4"() -> (w750:dbl[])
      n232 = local read "PWM8"() -> (w746:dbl[])
      n233 = local read "PWM5"() -> (w600:dbl[])
      n234 = local read "PWM6"() -> (w588:dbl[])
      n235 = local read "PWM5"() -> (w520:dbl[])
      n236 = local read "PWM4"() -> (w869:dbl[])
      n237 = local read "PWM8"() -> (w865:dbl[])
      n238 = local read "PWM7"() -> (w587:dbl[])
      n239 = local read "PWM6"() -> (w761:dbl[])
      n240 = local read "PWM6"() -> (w748:dbl[])
      n241 = local read "PWM1"() -> (w675:dbl[])
      n242 = local read "PWM1"() -> (w674:dbl[])
      n243 = local read "PWM3"() -> (w598:dbl[])
      n244 = local read "PWM3"() -> (w518:dbl[])
      n245 = local read "PWM6"() -> (w867:dbl[])
      n246 = local read "PWM7"() -> (w762:dbl[])
      n247 = local read "PWM7"() -> (w747:dbl[])
      n248 = local read "PWM4"() -> (w599:dbl[])
      n249 = local read "PWM8"() -> (w603:dbl[])
      n250 = local read "PWM4"() -> (w519:dbl[])
      n251 = local read "PWM8"() -> (w523:dbl[])
      n252 = local read "PWM7"() -> (w866:dbl[])
      n253 = local read "PWM9"() -> (w684:dbl[])
      n254 = local read "PWM9"() -> (w665:dbl[])
      n255 = local read "PWM6"() -> (w601:dbl[])
      n256 = local read "PWM6"() -> (w521:dbl[])
      n257 = local read "PWM7"() -> (w602:dbl[])
      n258 = local read "PWM7"() -> (w522:dbl[])
      n259 = local read "PWM2"() -> (w677:dbl[])
      n260 = local read "PWM2"() -> (w672:dbl[])
      n261 = local read "PWM5"() -> (w680:dbl[])
      n262 = local read "PWM5"() -> (w669:dbl[])
      n263 = local read "PWM3"() -> (w678:dbl[])
      n264 = local read "PWM3"() -> (w671:dbl[])
      n265 = local read "PWM4"() -> (w679:dbl[])
      n266 = local read "PWM8"() -> (w683:dbl[])
      n267 = local read "PWM4"() -> (w670:dbl[])
      n268 = local read "PWM8"() -> (w666:dbl[])
      n269 = local read "PWM6"() -> (w681:dbl[])
      n270 = local read "PWM6"() -> (w668:dbl[])
      n271 = local read "PWM7"() -> (w682:dbl[])
      n272 = local read "PWM7"() -> (w667:dbl[])
      n273 = Index Array(array=w874, index=w795) -> (element=w797:dbl)
      n274 = Index Array(array=w805, index=w795) -> (element=w823:dbl)
      n275 = Index Array(array=w594, index=w555) -> (element=w593:dbl)
      n276 = Index Array(array=w798, index=w795) -> (element=w816:dbl)
      n277 = Index Array(array=w755, index=w794) -> (element=w756:dbl)
      n278 = Index Array(array=w754, index=w715) -> (element=w753:dbl)
      n279 = Index Array(array=w585, index=w555) -> (element=w567:dbl)
      n280 = Index Array(array=w801, index=w795) -> (element=w819:dbl)
      n281 = Index Array(array=w873, index=w796) -> (element=w872:dbl)
      n282 = Index Array(array=w764, index=w794) -> (element=w782:dbl)
      n283 = Index Array(array=w745, index=w715) -> (element=w727:dbl)
      n284 = Index Array(array=w799, index=w795) -> (element=w817:dbl)
      n285 = Index Array(array=w864, index=w796) -> (element=w846:dbl)
      n286 = Index Array(array=w595, index=w634) -> (element=w596:dbl)
      n287 = Index Array(array=w592, index=w555) -> (element=w574:dbl)
      n288 = Index Array(array=w515, index=w554) -> (element=w516:dbl)
      n289 = Index Array(array=w800, index=w795) -> (element=w818:dbl)
      n290 = Index Array(array=w804, index=w795) -> (element=w822:dbl)
      n291 = Index Array(array=w757, index=w794) -> (element=w775:dbl)
      n292 = Index Array(array=w752, index=w715) -> (element=w734:dbl)
      n293 = Index Array(array=w604, index=w634) -> (element=w622:dbl)
      n294 = Index Array(array=w589, index=w555) -> (element=w571:dbl)
      n295 = Index Array(array=w524, index=w554) -> (element=w542:dbl)
      n296 = Index Array(array=w802, index=w795) -> (element=w820:dbl)
      n297 = Index Array(array=w871, index=w796) -> (element=w853:dbl)
      n298 = Index Array(array=w803, index=w795) -> (element=w821:dbl)
      n299 = Index Array(array=w760, index=w794) -> (element=w778:dbl)
      n300 = Index Array(array=w749, index=w715) -> (element=w731:dbl)
      n301 = Index Array(array=w591, index=w555) -> (element=w573:dbl)
      n302 = Index Array(array=w868, index=w796) -> (element=w850:dbl)
      n303 = Index Array(array=w597, index=w634) -> (element=w615:dbl)
      n304 = Index Array(array=w590, index=w555) -> (element=w572:dbl)
      n305 = Index Array(array=w586, index=w555) -> (element=w568:dbl)
      n306 = Index Array(array=w517, index=w554) -> (element=w535:dbl)
      n307 = Index Array(array=w758, index=w794) -> (element=w776:dbl)
      n308 = Index Array(array=w751, index=w715) -> (element=w733:dbl)
      n309 = Index Array(array=w870, index=w796) -> (element=w852:dbl)
      n310 = Index Array(array=w759, index=w794) -> (element=w777:dbl)
      n311 = Index Array(array=w763, index=w794) -> (element=w781:dbl)
      n312 = Index Array(array=w750, index=w715) -> (element=w732:dbl)
      n313 = Index Array(array=w746, index=w715) -> (element=w728:dbl)
      n314 = Index Array(array=w600, index=w634) -> (element=w618:dbl)
      n315 = Index Array(array=w588, index=w555) -> (element=w570:dbl)
      n316 = Index Array(array=w520, index=w554) -> (element=w538:dbl)
      n317 = Index Array(array=w869, index=w796) -> (element=w851:dbl)
      n318 = Index Array(array=w865, index=w796) -> (element=w847:dbl)
      n319 = Index Array(array=w587, index=w555) -> (element=w569:dbl)
      n320 = Index Array(array=w761, index=w794) -> (element=w779:dbl)
      n321 = Index Array(array=w748, index=w715) -> (element=w730:dbl)
      n322 = Index Array(array=w675, index=w714) -> (element=w676:dbl)
      n323 = Index Array(array=w674, index=w635) -> (element=w673:dbl)
      n324 = Index Array(array=w598, index=w634) -> (element=w616:dbl)
      n325 = Index Array(array=w518, index=w554) -> (element=w536:dbl)
      n326 = Index Array(array=w867, index=w796) -> (element=w849:dbl)
      n327 = Index Array(array=w762, index=w794) -> (element=w780:dbl)
      n328 = Index Array(array=w747, index=w715) -> (element=w729:dbl)
      n329 = Index Array(array=w599, index=w634) -> (element=w617:dbl)
      n330 = Index Array(array=w603, index=w634) -> (element=w621:dbl)
      n331 = Index Array(array=w519, index=w554) -> (element=w537:dbl)
      n332 = Index Array(array=w523, index=w554) -> (element=w541:dbl)
      n333 = Index Array(array=w866, index=w796) -> (element=w848:dbl)
      n334 = Index Array(array=w684, index=w714) -> (element=w702:dbl)
      n335 = Index Array(array=w665, index=w635) -> (element=w647:dbl)
      n336 = Index Array(array=w601, index=w634) -> (element=w619:dbl)
      n337 = Index Array(array=w521, index=w554) -> (element=w539:dbl)
      n338 = Index Array(array=w602, index=w634) -> (element=w620:dbl)
      n339 = Index Array(array=w522, index=w554) -> (element=w540:dbl)
      n340 = Index Array(array=w677, index=w714) -> (element=w695:dbl)
      n341 = Index Array(array=w672, index=w635) -> (element=w654:dbl)
      n342 = Index Array(array=w680, index=w714) -> (element=w698:dbl)
      n343 = Index Array(array=w669, index=w635) -> (element=w651:dbl)
      n344 = Index Array(array=w678, index=w714) -> (element=w696:dbl)
      n345 = Index Array(array=w671, index=w635) -> (element=w653:dbl)
      n346 = Index Array(array=w679, index=w714) -> (element=w697:dbl)
      n347 = Index Array(array=w683, index=w714) -> (element=w701:dbl)
      n348 = Index Array(array=w670, index=w635) -> (element=w652:dbl)
      n349 = Index Array(array=w666, index=w635) -> (element=w648:dbl)
      n350 = Index Array(array=w681, index=w714) -> (element=w699:dbl)
      n351 = Index Array(array=w668, index=w635) -> (element=w650:dbl)
      n352 = Index Array(array=w682, index=w714) -> (element=w700:dbl)
      n353 = Index Array(array=w667, index=w635) -> (element=w649:dbl)
      n354 = local read "PWM10"() -> (w814:dbl[])
      n355 = local read "PWM18"() -> (w806:dbl[])
      n356 = local read "PWM10"() -> (w576:dbl[])
      n357 = local read "PWM11"() -> (w813:dbl[])
      n358 = local read "PWM10"() -> (w773:dbl[])
      n359 = local read "PWM10"() -> (w736:dbl[])
      n360 = local read "PWM18"() -> (w584:dbl[])
      n361 = local read "PWM14"() -> (w810:dbl[])
      n362 = local read "PWM10"() -> (w855:dbl[])
      n363 = local read "PWM18"() -> (w765:dbl[])
      n364 = local read "PWM18"() -> (w744:dbl[])
      n365 = local read "PWM12"() -> (w812:dbl[])
      n366 = local read "PWM18"() -> (w863:dbl[])
      n367 = local read "PWM10"() -> (w613:dbl[])
      n368 = local read "PWM11"() -> (w577:dbl[])
      n369 = local read "PWM10"() -> (w533:dbl[])
      n370 = local read "PWM13"() -> (w811:dbl[])
      n371 = local read "PWM17"() -> (w807:dbl[])
      n372 = local read "PWM11"() -> (w772:dbl[])
      n373 = local read "PWM11"() -> (w737:dbl[])
      n374 = local read "PWM18"() -> (w605:dbl[])
      n375 = local read "PWM14"() -> (w580:dbl[])
      n376 = local read "PWM18"() -> (w525:dbl[])
      n377 = local read "PWM15"() -> (w809:dbl[])
      n378 = local read "PWM11"() -> (w856:dbl[])
      n379 = local read "PWM16"() -> (w808:dbl[])
      n380 = local read "PWM14"() -> (w769:dbl[])
      n381 = local read "PWM14"() -> (w740:dbl[])
      n382 = local read "PWM12"() -> (w578:dbl[])
      n383 = local read "PWM14"() -> (w859:dbl[])
      n384 = local read "PWM11"() -> (w612:dbl[])
      n385 = local read "PWM13"() -> (w579:dbl[])
      n386 = local read "PWM17"() -> (w583:dbl[])
      n387 = local read "PWM11"() -> (w532:dbl[])
      n388 = local read "PWM12"() -> (w771:dbl[])
      n389 = local read "PWM12"() -> (w738:dbl[])
      n390 = local read "PWM12"() -> (w857:dbl[])
      n391 = local read "PWM13"() -> (w770:dbl[])
      n392 = local read "PWM17"() -> (w766:dbl[])
      n393 = local read "PWM13"() -> (w739:dbl[])
      n394 = local read "PWM17"() -> (w743:dbl[])
      n395 = local read "PWM14"() -> (w609:dbl[])
      n396 = local read "PWM15"() -> (w581:dbl[])
      n397 = local read "PWM14"() -> (w529:dbl[])
      n398 = local read "PWM13"() -> (w858:dbl[])
      n399 = local read "PWM17"() -> (w862:dbl[])
      n400 = local read "PWM16"() -> (w582:dbl[])
      n401 = local read "PWM15"() -> (w768:dbl[])
      n402 = local read "PWM15"() -> (w741:dbl[])
      n403 = local read "PWM10"() -> (w693:dbl[])
      n404 = local read "PWM10"() -> (w656:dbl[])
      n405 = local read "PWM12"() -> (w611:dbl[])
      n406 = local read "PWM12"() -> (w531:dbl[])
      n407 = local read "PWM15"() -> (w860:dbl[])
      n408 = local read "PWM16"() -> (w767:dbl[])
      n409 = local read "PWM16"() -> (w742:dbl[])
      n410 = local read "PWM13"() -> (w610:dbl[])
      n411 = local read "PWM17"() -> (w606:dbl[])
      n412 = local read "PWM13"() -> (w530:dbl[])
      n413 = local read "PWM17"() -> (w526:dbl[])
      n414 = local read "PWM16"() -> (w861:dbl[])
      n415 = local read "PWM18"() -> (w685:dbl[])
      n416 = local read "PWM18"() -> (w664:dbl[])
      n417 = local read "PWM15"() -> (w608:dbl[])
      n418 = local read "PWM15"() -> (w528:dbl[])
      n419 = local read "PWM16"() -> (w607:dbl[])
      n420 = local read "PWM16"() -> (w527:dbl[])
      n421 = local read "PWM11"() -> (w692:dbl[])
      n422 = local read "PWM11"() -> (w657:dbl[])
      n423 = local read "PWM14"() -> (w689:dbl[])
      n424 = local read "PWM14"() -> (w660:dbl[])
      n425 = local read "PWM12"() -> (w691:dbl[])
      n426 = local read "PWM12"() -> (w658:dbl[])
      n427 = local read "PWM13"() -> (w690:dbl[])
      n428 = local read "PWM17"() -> (w686:dbl[])
      n429 = local read "PWM13"() -> (w659:dbl[])
      n430 = local read "PWM17"() -> (w663:dbl[])
      n431 = local read "PWM15"() -> (w688:dbl[])
      n432 = local read "PWM15"() -> (w661:dbl[])
      n433 = local read "PWM16"() -> (w687:dbl[])
      n434 = local read "PWM16"() -> (w662:dbl[])
      n435 = Index Array(array=w814, index=w795) -> (element=w824:dbl)
      n436 = Index Array(array=w806, index=w795) -> (element=w832:dbl)
      n437 = Index Array(array=w576, index=w555) -> (element=w566:dbl)
      n438 = Index Array(array=w813, index=w795) -> (element=w825:dbl)
      n439 = Index Array(array=w773, index=w794) -> (element=w783:dbl)
      n440 = Index Array(array=w736, index=w715) -> (element=w726:dbl)
      n441 = Index Array(array=w584, index=w555) -> (element=w558:dbl)
      n442 = Index Array(array=w810, index=w795) -> (element=w828:dbl)
      n443 = Index Array(array=w855, index=w796) -> (element=w845:dbl)
      n444 = Index Array(array=w765, index=w794) -> (element=w791:dbl)
      n445 = Index Array(array=w744, index=w715) -> (element=w718:dbl)
      n446 = Index Array(array=w812, index=w795) -> (element=w826:dbl)
      n447 = Index Array(array=w863, index=w796) -> (element=w837:dbl)
      n448 = Index Array(array=w613, index=w634) -> (element=w623:dbl)
      n449 = Index Array(array=w577, index=w555) -> (element=w565:dbl)
      n450 = Index Array(array=w533, index=w554) -> (element=w543:dbl)
      n451 = Index Array(array=w811, index=w795) -> (element=w827:dbl)
      n452 = Index Array(array=w807, index=w795) -> (element=w831:dbl)
      n453 = Index Array(array=w772, index=w794) -> (element=w784:dbl)
      n454 = Index Array(array=w737, index=w715) -> (element=w725:dbl)
      n455 = Index Array(array=w605, index=w634) -> (element=w631:dbl)
      n456 = Index Array(array=w580, index=w555) -> (element=w562:dbl)
      n457 = Index Array(array=w525, index=w554) -> (element=w551:dbl)
      n458 = Index Array(array=w809, index=w795) -> (element=w829:dbl)
      n459 = Index Array(array=w856, index=w796) -> (element=w844:dbl)
      n460 = Index Array(array=w808, index=w795) -> (element=w830:dbl)
      n461 = Index Array(array=w769, index=w794) -> (element=w787:dbl)
      n462 = Index Array(array=w740, index=w715) -> (element=w722:dbl)
      n463 = Index Array(array=w578, index=w555) -> (element=w564:dbl)
      n464 = Index Array(array=w859, index=w796) -> (element=w841:dbl)
      n465 = Index Array(array=w612, index=w634) -> (element=w624:dbl)
      n466 = Index Array(array=w579, index=w555) -> (element=w563:dbl)
      n467 = Index Array(array=w583, index=w555) -> (element=w559:dbl)
      n468 = Index Array(array=w532, index=w554) -> (element=w544:dbl)
      n469 = Index Array(array=w771, index=w794) -> (element=w785:dbl)
      n470 = Index Array(array=w738, index=w715) -> (element=w724:dbl)
      n471 = Index Array(array=w857, index=w796) -> (element=w843:dbl)
      n472 = Index Array(array=w770, index=w794) -> (element=w786:dbl)
      n473 = Index Array(array=w766, index=w794) -> (element=w790:dbl)
      n474 = Index Array(array=w739, index=w715) -> (element=w723:dbl)
      n475 = Index Array(array=w743, index=w715) -> (element=w719:dbl)
      n476 = Index Array(array=w609, index=w634) -> (element=w627:dbl)
      n477 = Index Array(array=w581, index=w555) -> (element=w561:dbl)
      n478 = Index Array(array=w529, index=w554) -> (element=w547:dbl)
      n479 = Index Array(array=w858, index=w796) -> (element=w842:dbl)
      n480 = Index Array(array=w862, index=w796) -> (element=w838:dbl)
      n481 = Index Array(array=w582, index=w555) -> (element=w560:dbl)
      n482 = Index Array(array=w768, index=w794) -> (element=w788:dbl)
      n483 = Index Array(array=w741, index=w715) -> (element=w721:dbl)
      n484 = Index Array(array=w693, index=w714) -> (element=w703:dbl)
      n485 = Index Array(array=w656, index=w635) -> (element=w646:dbl)
      n486 = Index Array(array=w611, index=w634) -> (element=w625:dbl)
      n487 = Index Array(array=w531, index=w554) -> (element=w545:dbl)
      n488 = Index Array(array=w860, index=w796) -> (element=w840:dbl)
      n489 = Index Array(array=w767, index=w794) -> (element=w789:dbl)
      n490 = Index Array(array=w742, index=w715) -> (element=w720:dbl)
      n491 = Index Array(array=w610, index=w634) -> (element=w626:dbl)
      n492 = Index Array(array=w606, index=w634) -> (element=w630:dbl)
      n493 = Index Array(array=w530, index=w554) -> (element=w546:dbl)
      n494 = Index Array(array=w526, index=w554) -> (element=w550:dbl)
      n495 = Index Array(array=w861, index=w796) -> (element=w839:dbl)
      n496 = Index Array(array=w685, index=w714) -> (element=w711:dbl)
      n497 = Index Array(array=w664, index=w635) -> (element=w638:dbl)
      n498 = Index Array(array=w608, index=w634) -> (element=w628:dbl)
      n499 = Index Array(array=w528, index=w554) -> (element=w548:dbl)
      n500 = Index Array(array=w607, index=w634) -> (element=w629:dbl)
      n501 = Index Array(array=w527, index=w554) -> (element=w549:dbl)
      n502 = Index Array(array=w692, index=w714) -> (element=w704:dbl)
      n503 = Index Array(array=w657, index=w635) -> (element=w645:dbl)
      n504 = Index Array(array=w689, index=w714) -> (element=w707:dbl)
      n505 = Index Array(array=w660, index=w635) -> (element=w642:dbl)
      n506 = Index Array(array=w691, index=w714) -> (element=w705:dbl)
      n507 = Index Array(array=w658, index=w635) -> (element=w644:dbl)
      n508 = Index Array(array=w690, index=w714) -> (element=w706:dbl)
      n509 = Index Array(array=w686, index=w714) -> (element=w710:dbl)
      n510 = Index Array(array=w659, index=w635) -> (element=w643:dbl)
      n511 = Index Array(array=w663, index=w635) -> (element=w639:dbl)
      n512 = Index Array(array=w688, index=w714) -> (element=w708:dbl)
      n513 = Index Array(array=w661, index=w635) -> (element=w641:dbl)
      n514 = Index Array(array=w687, index=w714) -> (element=w709:dbl)
      n515 = Index Array(array=w662, index=w635) -> (element=w640:dbl)
      n516 = local read "PWM19"() -> (w815:dbl[])
      n517 = local read "PWM19"() -> (w575:dbl[])
      n518 = local read "PWM19"() -> (w774:dbl[])
      n519 = local read "PWM19"() -> (w735:dbl[])
      n520 = local read "PWM19"() -> (w854:dbl[])
      n521 = local read "PWM19"() -> (w614:dbl[])
      n522 = local read "PWM19"() -> (w534:dbl[])
      n523 = local read "PWM19"() -> (w694:dbl[])
      n524 = local read "PWM19"() -> (w655:dbl[])
      n525 = Index Array(array=w815, index=w795) -> (element=w833:dbl)
      n526 = Index Array(array=w575, index=w555) -> (element=w557:dbl)
      n527 = Index Array(array=w774, index=w794) -> (element=w792:dbl)
      n528 = Index Array(array=w735, index=w715) -> (element=w717:dbl)
      n529 = Index Array(array=w854, index=w796) -> (element=w836:dbl)
      n530 = Index Array(array=w614, index=w634) -> (element=w632:dbl)
      n531 = Index Array(array=w534, index=w554) -> (element=w552:dbl)
      n532 = Index Array(array=w694, index=w714) -> (element=w712:dbl)
      n533 = Index Array(array=w655, index=w635) -> (element=w637:dbl)
      n534 = Build Array(w797, w816, w817, w818, w819, w820, w821, w822, w823, w824, w825, w826, w827, w828, w829, w830, w831, w832, w833) -> (→"SENSOR1":dbl[])
      n535 = Build Array(w593, w574, w573, w572, w571, w570, w569, w568, w567, w566, w565, w564, w563, w562, w561, w560, w559, w558, w557) -> (→"SENSOR 8":dbl[])
      n536 = Build Array(w756, w775, w776, w777, w778, w779, w780, w781, w782, w783, w784, w785, w786, w787, w788, w789, w790, w791, w792) -> (→"SENSOR 3":dbl[])
      n537 = Build Array(w753, w734, w733, w732, w731, w730, w729, w728, w727, w726, w725, w724, w723, w722, w721, w720, w719, w718, w717) -> (→"SENSOR 4":dbl[])
      n538 = Build Array(w872, w853, w852, w851, w850, w849, w848, w847, w846, w845, w844, w843, w842, w841, w840, w839, w838, w837, w836) -> (→"SENSOR 2":dbl[])
      n539 = Build Array(w596, w615, w616, w617, w618, w619, w620, w621, w622, w623, w624, w625, w626, w627, w628, w629, w630, w631, w632) -> (→"SENSOR 7":dbl[])
      n540 = Build Array(w516, w535, w536, w537, w538, w539, w540, w541, w542, w543, w544, w545, w546, w547, w548, w549, w550, w551, w552) -> (→"SENSOR 9":dbl[])
      n541 = Build Array(w676, w695, w696, w697, w698, w699, w700, w701, w702, w703, w704, w705, w706, w707, w708, w709, w710, w711, w712) -> (→"SENSOR 5":dbl[])
      n542 = Build Array(w673, w654, w653, w652, w651, w650, w649, w648, w647, w646, w645, w644, w643, w642, w641, w640, w639, w638, w637) -> (→"SENSOR 6":dbl[])
    }
  }
